vi "acquireSpectraWithOverSaturationProtection.vi"(8 "error in (no error)":errorcluster, 9 "NumberOfAcquisitions (1)":i32=1, 10 "default_integration_time":i32, 11 "VISA_name":refnum<visa-resource-name>) -> (0 "error out":errorcluster, 2 "integration_time":i32, 3 "Spectrum":dbl[](array[numeric]))   [LabVIEW 2015]
uses:
  <instrlib>/Ocean Optics 2000 4000/Ocean Optics 2000 4000.lvlib
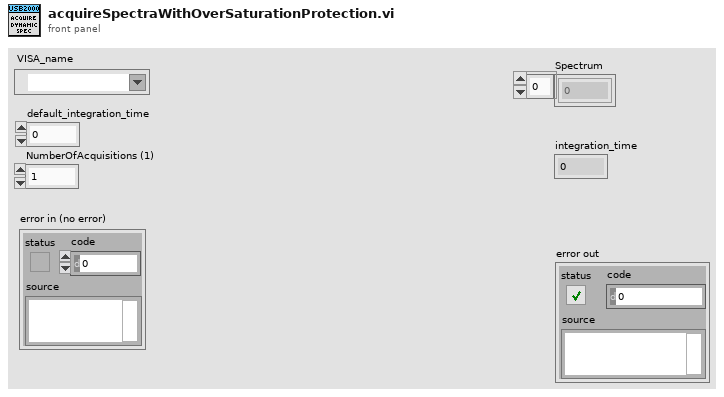
[diagram p1: front panel]
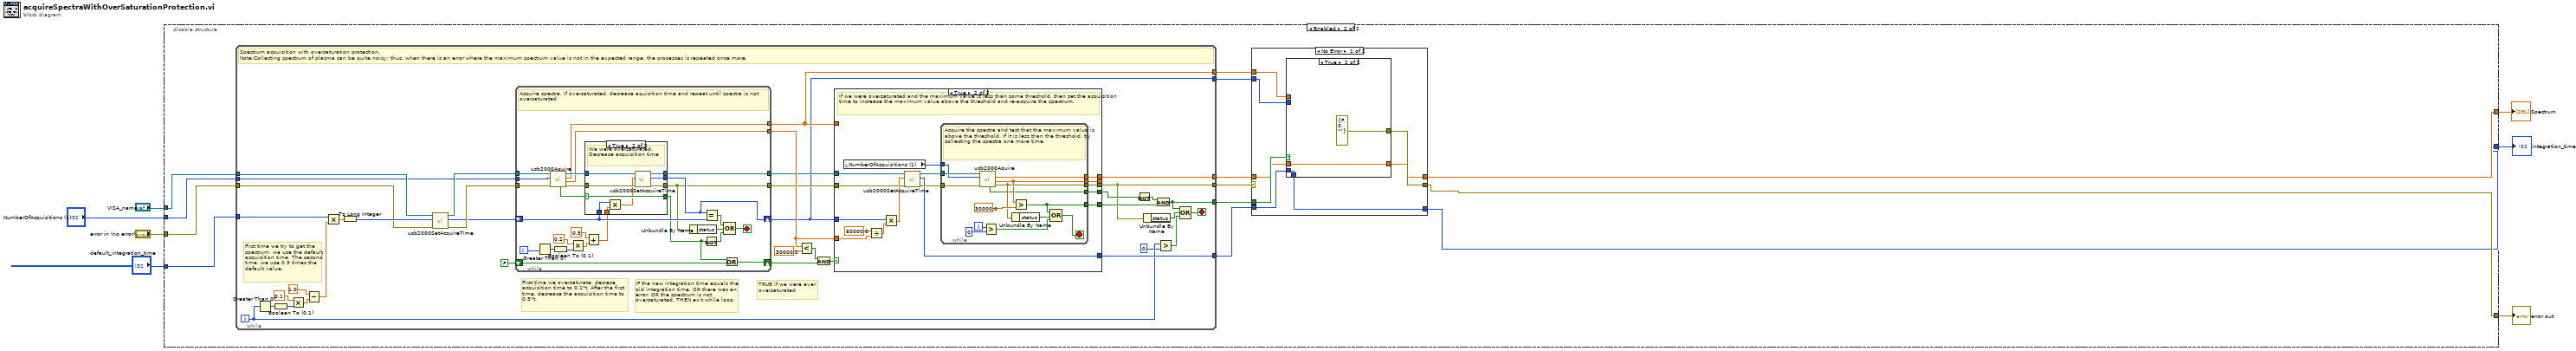
[diagram p0: block diagram]
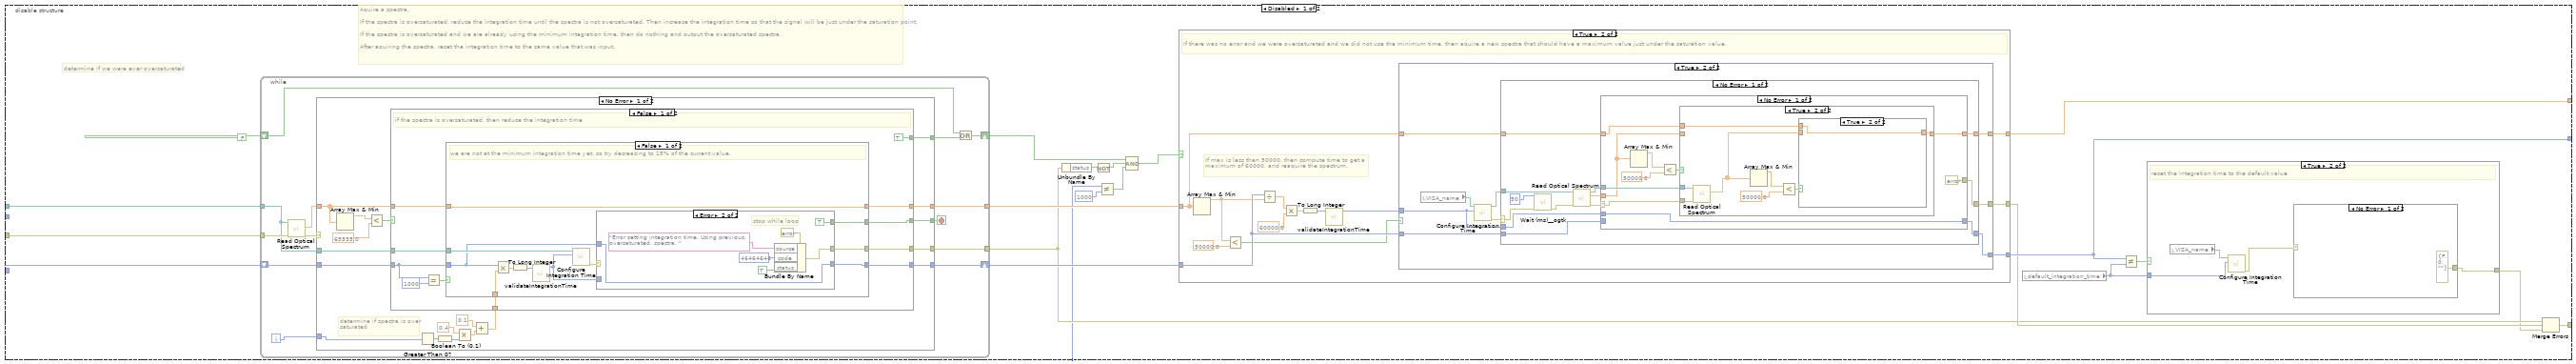
[diagram p2: hidden frame]
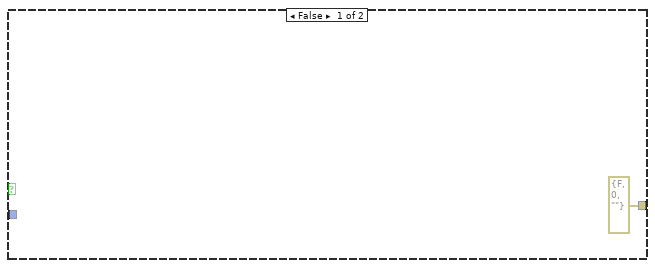
[diagram p3: hidden frame]
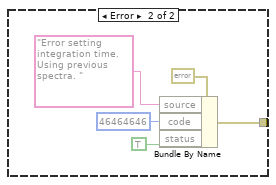
[diagram p4: hidden frame]
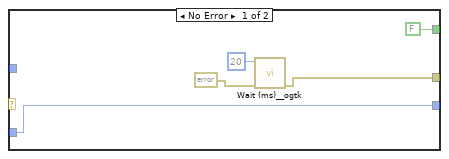
[diagram p5: hidden frame]
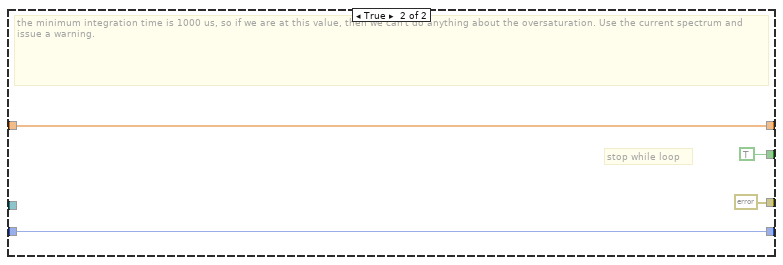
[diagram p6: hidden frame]
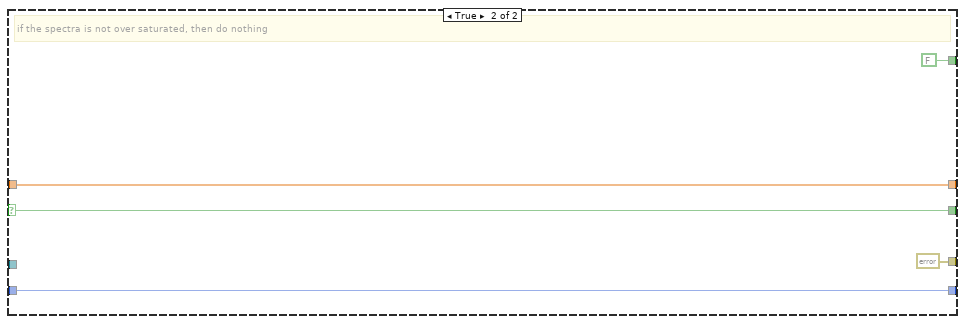
[diagram p7: hidden frame]
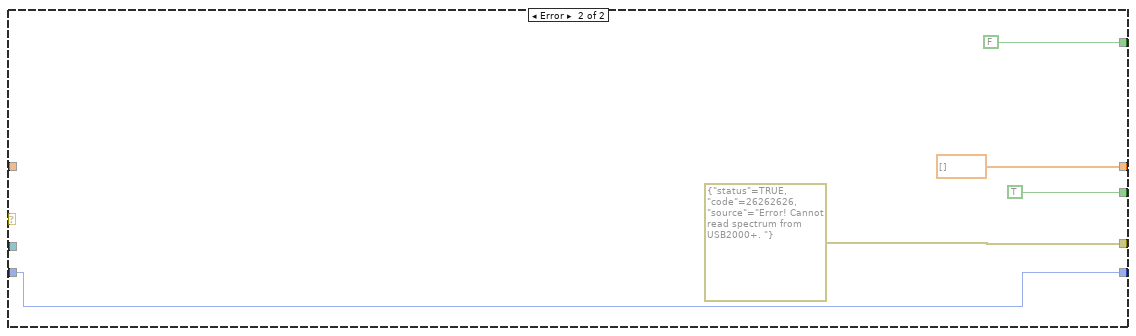
[diagram p8: hidden frame]
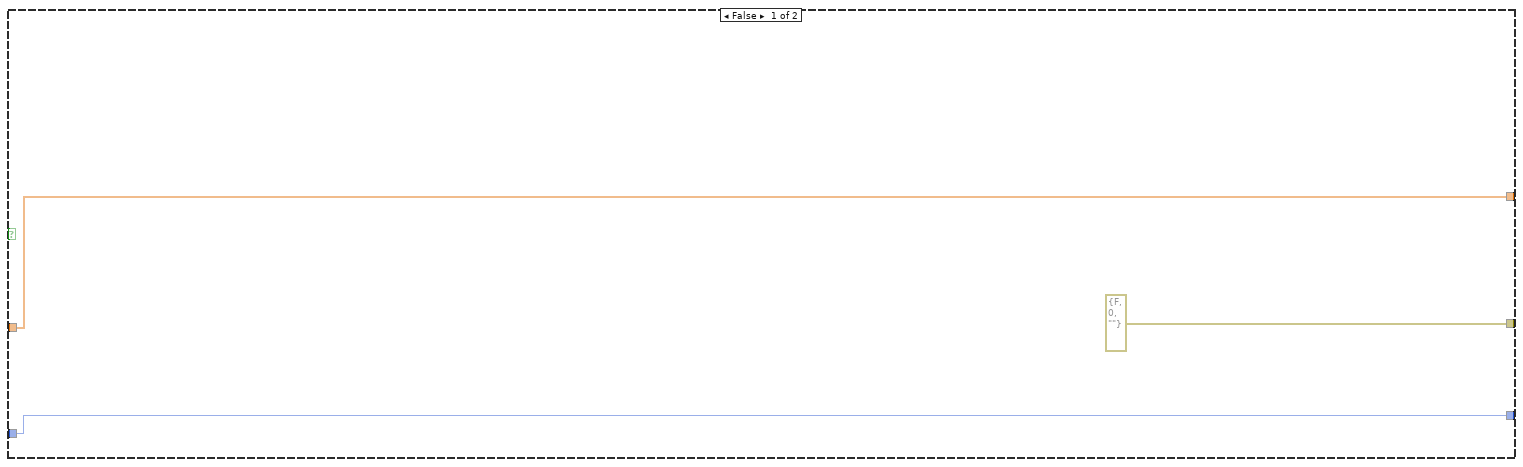
[diagram p9: hidden frame]
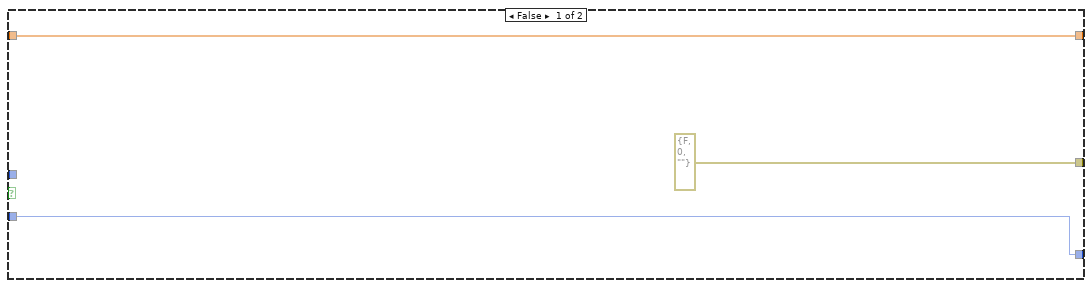
[diagram p10: hidden frame]
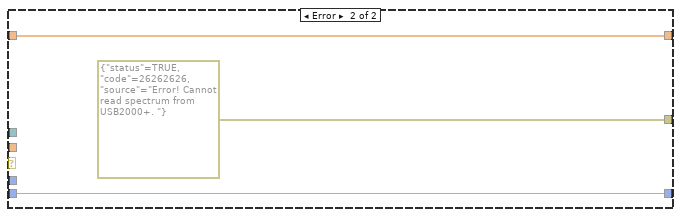
[diagram p13: hidden frame]
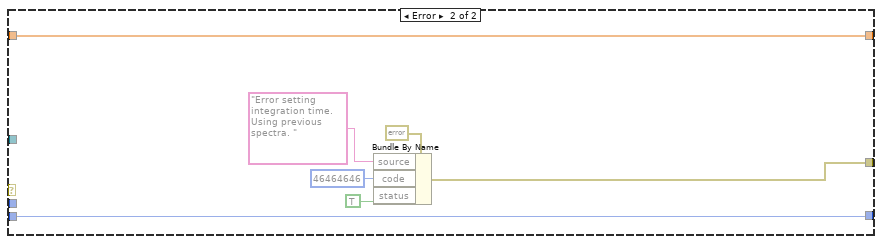
[diagram p14: hidden frame]
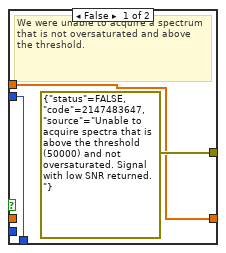
[diagram p15: hidden frame]
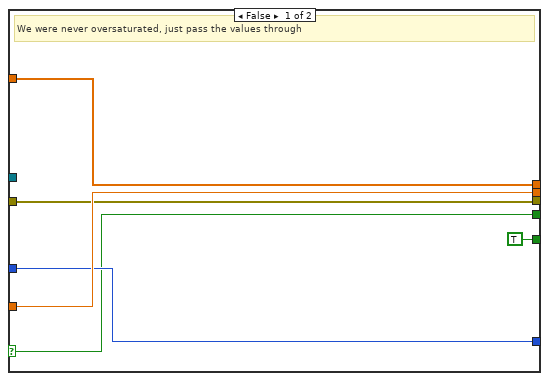
[diagram p17: hidden frame]
diagram:
  n1 = disable-structure shown="Enabled" {
    disable-tunnel: "error in (no error)" -> [w27 w198]
    disable-tunnel: [w19 w192] -> w6
    disable-tunnel: [w15 w194] -> w5
    disable-tunnel: [w14 w196] -> w4
    disable-tunnel: "default_integration_time" -> [w9 w199]
    disable-tunnel: "VISA_name" -> [w8 w197]
    disable-tunnel: "NumberOfAcquisitions (1)" -> [_ w195]
    frame Disabled {
      # "Aquire a spectra.\n\nIf the spectra is oversaturated, reduce the integration time until the spectra is not oversaturated. Then increase the integration time so that the signal will be just under the saturation point.\n\nIf the spectra is oversaturated and we are already using the minimum integration time, then do nothing and output the oversaturated spectra.\n\nAfter aquiring the spectra, reset the integration time to the same value that was input."
      # "determine if we were ever oversaturated"
      n2 = while {
        tunnel: w27 -> [w41]
        tunnel: w8 -> [w40]
        shift-right: [w49] -> w24
        shift-left: FALSE -> [w45]
        shift-right: [w48] -> w21
        shift-left: w9 -> [w51]
        tunnel: [w47] -> w20
        tunnel: [w44] -> w13
        i -> [w43]
        stop <- w50 stop-if-true
        n3 = call <instrlib>:"Read Optical Spectrum.vi"("error in (no error)"=w41, "VISA resource name"=w40) -> ("error out"=w39:errorcluster, "Spectrum by Pixels"=w42:dbl[])  [unwired: 6 in, 2 out]
        n4 = case shown="No Error" w39 {
          tunnel: w42 -> [w61 _]
          tunnel: [w62 errorcluster {"status"=TRUE, "code"=26262626, "source"="Error! Cannot read spectrum from USB2000+. "} ("error constant")] -> w44
          tunnel: [w68 dbl[] [] ("Spectrum by Pixels")] -> w47
          tunnel: w51 -> [w67 w115]
          tunnel: [w66 w115] -> w48
          tunnel: w40 -> [w65 _]
          tunnel: [w64 TRUE] -> w50
          tunnel: [w63 FALSE] -> w46
          tunnel: w43 -> [w58 _]
          frame No Error {
            # "determine if spectra is over saturated"
            n5 = Array Max & Min(array=w61) -> (max value=w60:dbl)  [unwired: 3 out]
            n6 = Less?(x=w60, y=65535.0) -> (x < y?=w59:bool)
            n7 = Greater Than 0?(x=w58) -> (x > 0?=w57:bool)
            n8 = Boolean To (0,1)(Boolean=w57) -> (0, 1=w56:i16)
            n9 = Multiply(x=0.4, y=w56) -> (x*y=w54:dbl)
            n10 = Add(x=0.1, y=w54) -> (x+y=w52:dbl)
            n11 = case shown="False" w59 {
              selector: w59 -> [_ w111]
              tunnel: w61 -> [w80 w112]
              tunnel: [w79 w112] -> w68
              tunnel: w67 -> [w72 w109]
              tunnel: [w78 w109] -> w66
              tunnel: w65 -> [w75 _]
              tunnel: [w77 w111] -> w64
              tunnel: [TRUE FALSE] -> w63
              tunnel: [w74 errorcluster {"status"=FALSE, "code"=0, "source"=""} ("error constant")] -> w62
              tunnel: w52 -> [w70 _]
              frame False {
                # "if the spectra is oversaturated, then reduce the integration time"
                n12 = Equal?(x=w72, y=1000) -> (x = y?=w73:bool)
                n13 = case shown="False" w73 {
                  tunnel: w80 -> [w89 w107]
                  tunnel: [w89 w107] -> w79
                  tunnel: w72 -> [w85 w106]
                  tunnel: [w86 w106] -> w78
                  tunnel: [w87 TRUE] -> w77
                  tunnel: w75 -> [w90 _]
                  tunnel: [w84 errorcluster {"status"=FALSE, "code"=0, "source"=""} ("error constant")] -> w74
                  tunnel: w70 -> [w81 _]
                  frame False {
                    # "we are not at the minimum integration time yet, so try decreasing to 15% of the current value."
                    n14 = Multiply(x=w85, y=w81) -> (x*y=w91:dbl)
                    n15 = To Long Integer(number=w91) -> (32bit integer=w83:i32)
                    n16 = call "validateIntegrationTime.vi"("integrationTime"=w83) -> ("validIntegrationTime"=w82:i32)  [unwired: 10 in]
                    n17 = call <instrlib>:"Configure Integration Time.vi"("Integration Time (6000)"=w82, "VISA resource name"=w90) -> ("error out"=w88:errorcluster)  [unwired: 1 in, 8 out]
                    n18 = case shown="Error" w88 {
                      tunnel: [FALSE TRUE] -> w87
                      tunnel: w82 -> [w95 _]
                      tunnel: [w95 w98] -> w86
                      tunnel: w85 -> [_ w98]
                      tunnel: [w93 w100] -> w84
                      frame No Error {
                        n19 = call <userlib>:"Wait (ms)__ogtk.vi"("error in (no error)"=errorcluster {"status"=FALSE, "code"=0, "source"=""} ("error constant"), "milliseconds to wait"=u32 20) -> ("error out"=w93:errorcluster)  [unwired: 8 in, 1 out]
                      }
                      frame Error {
                        # "stop while loop"
                        n20 = Bundle By Name(cluster=errorcluster {"status"=FALSE, "code"=0, "source"=""} ("error constant"), "source"="Error setting integration time. Using previous, oversaturated, spectra. ", "code"=46464646, "status"=TRUE) -> (w100:errorcluster)
                      }
                    }
                  }
                  frame True {
                    # "stop while loop"
                    # "the minimum integration time is 1000 us, so if we are at this value, then we can't do anything about the oversaturation. Use the current spectrum and issue a warning."
                  }
                }
              }
              frame True {
                # "if the spectra is not over saturated, then do nothing"
              }
            }
          }
          frame Error {
          }
        }
        n21 = Or(x=w45, y=w46) -> (x .or. y?=w49:bool)
      }
      n22 = Unbundle By Name(w13) -> ("status"=w25:bool)
      n23 = Not(x=w25) -> (.not. x?=w23:bool)
      n24 = Not Equal?(x=w9, y=1000) -> (x != y?=w10:bool)
      n25 = Compound Arithmetic op=AND(w24, w23, w10) -> (w22:bool)
      n26 = case shown="True" w22 {
        tunnel: w21 -> [w119 w128]
        tunnel: w20 -> [w120 w131]
        tunnel: [w120 w130] -> w14
        tunnel: [w119 w129] -> w19
        tunnel: [errorcluster {"status"=FALSE, "code"=0, "source"=""} ("error constant") w127] -> w16
        frame False {
        }
        frame True {
          # "If max is less than 50000, then compute time to get a maximum of 60000, and reaquire the spectrum."
          # "If there was no error and we were oversaturated and we did not use the minimum time, then aquire a new spectra that should have a maximum value just under the saturation value."
          n27 = Array Max & Min(array=w131) -> (max value=w123:dbl)  [unwired: 3 out]
          n28 = Less?(x=w123, y=50000.0) -> (x < y?=w121:bool)
          n29 = Divide(x=w128, y=w123) -> (x/y=w133:dbl)
          n30 = Multiply(x=w133, y=60000.0) -> (x*y=w132:dbl)
          n31 = To Long Integer(number=w132) -> (32bit integer=w125:i32)
          n32 = call "validateIntegrationTime.vi"("integrationTime"=w125) -> ("validIntegrationTime"=w124:i32)  [unwired: 10 in]
          n33 = case shown="True" w121 {
            tunnel: w124 -> [_ w139]
            tunnel: w131 -> [w136 w143]
            tunnel: [w136 w142] -> w130
            tunnel: [w135 w140] -> w129
            tunnel: w128 -> [w135 w137]
            tunnel: [errorcluster {"status"=FALSE, "code"=0, "source"=""} ("error constant") w141] -> w127
            frame False {
            }
            frame True {
              n34 = local read "VISA_name"() -> (w144:refnum<visa-resource-name>)
              n35 = call <instrlib>:"Configure Integration Time.vi"("Integration Time (6000)"=w139, "VISA resource name"=w144) -> ("error out"=w145:errorcluster, "VISA resource name out"=w138:refnum<visa-resource-name>)  [unwired: 1 in, 7 out]
              n36 = case shown="No Error" w145 {
                selector: w145 -> [w152 _]
                tunnel: [w156 w187] -> w141
                tunnel: w138 -> [w150 _]
                tunnel: w143 -> [w157 w184]
                tunnel: [w158 w184] -> w142
                tunnel: w139 -> [w155 _]
                tunnel: [w153 w183] -> w140
                tunnel: w137 -> [w154 w183]
                frame No Error {
                  n37 = call <userlib>:"Wait (ms)__ogtk.vi"("error in (no error)"=w152, "milliseconds to wait"=u32 50) -> ("error out"=w149:errorcluster)  [unwired: 8 in, 1 out]
                  n38 = call <instrlib>:"Read Optical Spectrum.vi"("error in (no error)"=w149, "VISA resource name"=w150) -> ("error out"=w147:errorcluster, "Spectrum by Pixels"=w148:dbl[], "VISA resource name out"=w146:refnum<visa-resource-name>)  [unwired: 6 in, 1 out]
                  n39 = case shown="No Error" w147 {
                    selector: w147 -> [w163 _]
                    tunnel: w148 -> [w161 _]
                    tunnel: [w160 w182] -> w158
                    tunnel: w157 -> [w159 w182]
                    tunnel: [errorcluster {"status"=FALSE, "code"=0, "source"=""} ("error constant") errorcluster {"status"=TRUE, "code"=26262626, "source"="Error! Cannot read spectrum from USB2000+. "} ("error constant")] -> w156
                    tunnel: w155 -> [w167 _]
                    tunnel: w154 -> [_ w180]
                    tunnel: [w167 w180] -> w153
                    tunnel: w146 -> [w162 _]
                    frame No Error {
                      n40 = Array Max & Min(array=w161) -> (max value=w166:dbl)  [unwired: 3 out]
                      n41 = Less?(x=w166, y=50000.0) -> (x < y?=w164:bool)
                      n42 = case shown="True" w164 {
                        tunnel: w163 -> [_ w177]
                        tunnel: w162 -> [_ w176]
                        tunnel: w161 -> [w169 _]
                        tunnel: [w169 w171] -> w160
                        tunnel: w159 -> [_ w170]
                        frame False {
                        }
                        frame True {
                          n43 = call <instrlib>:"Read Optical Spectrum.vi"("error in (no error)"=w177, "VISA resource name"=w176) -> ("Spectrum by Pixels"=w172:dbl[])  [unwired: 6 in, 3 out]
                          n44 = Array Max & Min(array=w172) -> (max value=w174:dbl)  [unwired: 3 out]
                          n45 = Less?(x=w174, y=50000.0) -> (x < y?=w173:bool)
                          n46 = case shown="True" w173 {
                            tunnel: w172 -> [w178 _]
                            tunnel: [w178 w179] -> w171
                            tunnel: w170 -> [_ w179]
                            frame False {
                            }
                            frame True {
                            }
                          }
                        }
                      }
                    }
                    frame Error {
                    }
                  }
                }
                frame Error {
                  n47 = Bundle By Name(cluster=errorcluster {"status"=FALSE, "code"=0, "source"=""} ("error constant"), "source"="Error setting integration time. Using previous spectra. ", "code"=46464646, "status"=TRUE) -> (w187:errorcluster)
                }
              }
            }
          }
        }
      }
      n48 = local read "default_integration_time"() -> (w17:i32)
      n49 = Not Equal?(x=w19, y=w17) -> (x != y?=w18:bool)
      n50 = case shown="True" w18 {
        tunnel: w17 -> [_ w31]
        tunnel: [errorcluster {"status"=FALSE, "code"=0, "source"=""} ("error constant") w29] -> w12
        frame False {
        }
        frame True {
          # "reset the integration time to the default value"
          n51 = local read "VISA_name"() -> (w32:refnum<visa-resource-name>)
          n52 = call <instrlib>:"Configure Integration Time.vi"("Integration Time (6000)"=w31, "VISA resource name"=w32) -> ("error out"=w30:errorcluster)  [unwired: 1 in, 8 out]
          n53 = case shown="No Error" w30 {
            tunnel: [errorcluster {"status"=FALSE, "code"=0, "source"=""} ("error constant") w34] -> w29
            frame No Error {
            }
            frame Error {
              n54 = Bundle By Name(cluster=errorcluster {"status"=FALSE, "code"=0, "source"=""} ("error constant"), "source"="Error setting integration time. Using previous spectra. ", "code"=46464646, "status"=TRUE) -> (w34:errorcluster)
            }
          }
        }
      }
      n55 = Merge Errors(w13, w16, w12) -> (w15:errorcluster)
    }
    frame Enabled {
      n56 = while {
        tunnel: w199 -> [w233]
        tunnel: [w241] -> w202
        tunnel: [w240] -> w200
        tunnel: [w239] -> w193
        tunnel: [w231] -> w201
        tunnel: w197 -> [w224]
        tunnel: w198 -> [w223]
        tunnel: w195 -> [w222]
        tunnel: [w221] -> w191
        tunnel: [w220] -> w190
        i -> [w234]
        stop <- w242 stop-if-true
        # "First time we try to get the spectrum, we use the default acquisition time. The second time, we use 0.9 times the default value."
        # "IF the new integration time equals the old integration time, OR there was an error, OR the spectrum is not oversaturated, THEN exit while loop"
        # "First time we oversaturate, decrese acquisition time to 0.1*t. After the first time, decrease the acquisition time to 0.5*t."
        # "TRUE if we were ever oversaturated"
        # "Spectrum acquisition with oversaturation protection. \nNote:Collecting spectrum of plasma can be quite noisy; thus, when there is an error where the maximum spectrum value is not in the expected range, the processes is repeated once more."
        n57 = Greater Than 0?(x=w234) -> (x > 0?=w229:bool)
        n58 = Boolean To (0,1)(Boolean=w229) -> (0, 1=w238:i16)
        n59 = Multiply(x=0.1, y=w238) -> (x*y=w236:dbl)
        n60 = Subtract(x=1.0, y=w236) -> (x-y=w232:dbl)
        n61 = Multiply(x=w233, y=w232) -> (x*y=w230:dbl)
        n62 = To Long Integer(number=w230) -> (32bit integer=w225:i32)
        n63 = call "usb2000SetAcquireTime.vi"("error in (no error)"=w223, "Integration Time (6000)"=w225, "VISA resource name"=w224) -> ("error out"=w227:errorcluster, "validIntegrationTime"=w226:i32, "VISA resource name out"=w228:refnum<visa-resource-name>)  [unwired: 6 in]
        n64 = while {
          shift-right: [w303] -> w220
          shift-left: w226 -> [w309]
          tunnel: [w302] -> w221
          tunnel: [w301] -> w251
          shift-right: [w300] -> w252
          shift-left: FALSE -> [w298]
          tunnel: [w297] -> w250
          tunnel: [w296] -> w249
          tunnel: w228 -> [w295]
          tunnel: w227 -> [w294]
          tunnel: w222 -> [w293]
          i -> [w310]
          stop <- w304 stop-if-true
          # "Acquire spectra. If oversaturated, decrease aquisition time and repeat until spectra is not oversaturated"
          n65 = Greater Than 0?(x=w310) -> (x > 0?=w311:bool)
          n66 = call "usb2000Aquire.vi"("error in (no error)"=w294, "NumberOfAcquisitions (1)"=w293, "VISA resource name"=w295) -> ("error out"=w317:errorcluster, "MaxValue"=w301:dbl, "Spectrum by Pixels"=w302:dbl[], "VISA resource name out"=w316:refnum<visa-resource-name>, "oversaturated"=w318:bool)  [unwired: 4 in]
          n67 = Boolean To (0,1)(Boolean=w311) -> (0, 1=w312:i16)
          n68 = Multiply(x=0.2, y=w312) -> (x*y=w314:dbl)
          n69 = Add(x=0.5, y=w314) -> (x+y=w308:dbl)
          n70 = case shown="True" w318 {
            selector: w318 -> [w322 w328]
            tunnel: w317 -> [w321 w331]
            tunnel: w316 -> [w319 w330]
            tunnel: [w321 w329] -> w297
            tunnel: [w322 w328] -> w299
            tunnel: [w320 w327] -> w303
            tunnel: w309 -> [w320 w326]
            tunnel: w308 -> [_ w325]
            tunnel: [w319 w323] -> w296
            frame False {
            }
            frame True {
              # "We were oversaturated. Decrease acquisition time"
              n71 = Multiply(x=w326, y=w325) -> (x*y=w324:dbl)
              n72 = call "usb2000SetAcquireTime.vi"("error in (no error)"=w331, "Integration Time (6000)"=w324, "VISA resource name"=w330) -> ("error out"=w329:errorcluster, "validIntegrationTime"=w327:i32, "VISA resource name out"=w323:refnum<visa-resource-name>)  [unwired: 6 in]
            }
          }
          n73 = Unbundle By Name(w297) -> ("status"=w306:bool)
          n74 = Not(x=w299) -> (.not. x?=w305:bool)
          n75 = Equal?(x=w303, y=w309) -> (x = y?=w307:bool)
          n76 = Compound Arithmetic op=OR(w307, w306, w305) -> (w304:bool)
          n77 = Or(x=w299, y=w298) -> (x .or. y?=w300:bool)
        }
        n78 = Less?(x=w251, y=30000.0) -> (x < y?=w253:bool)
        n79 = And(x=w253, y=w252) -> (x .and. y?=w254:bool)
        n80 = case shown="True" w254 {
          selector: w254 -> [w257 _]
          tunnel: w220 -> [w259 w278]
          tunnel: w251 -> [w261 w275]
          tunnel: w250 -> [w260 w274]
          tunnel: w249 -> [_ w272]
          tunnel: [w259 w269] -> w239
          tunnel: [w260 w266] -> w240
          tunnel: [w261 w268] -> _
          tunnel: [w262 w267] -> w241
          tunnel: w221 -> [w262 _]
          tunnel: [w257 w265] -> w245
          tunnel: [TRUE w264] -> w246
          frame False {
            # "We were never oversaturated, just pass the values through"
          }
          frame True {
            # "If we were oversaturated and the maximum value is less than some threshold, then set the acquisition time to increase the maximum value above the threshold and re-acquire the spectrum."
            n81 = local read "NumberOfAcquisitions (1)"() -> (w263:i32)
            n82 = Divide(x=60000.0, y=w275) -> (x/y=w277:dbl)
            n83 = Multiply(x=w278, y=w277) -> (x*y=w273:dbl)
            n84 = call "usb2000SetAcquireTime.vi"("error in (no error)"=w274, "Integration Time (6000)"=w273, "VISA resource name"=w272) -> ("error out"=w271:errorcluster, "validIntegrationTime"=w269:i32, "VISA resource name out"=w270:refnum<visa-resource-name>)  [unwired: 6 in]
            n85 = while {
              tunnel: w271 -> [w292]
              tunnel: w270 -> [w291]
              tunnel: [w287] -> w267
              tunnel: [w283] -> w266
              tunnel: [w282] -> w268
              tunnel: [w281] -> w265
              tunnel: [w280] -> w264
              tunnel: w263 -> [w279]
              i -> [w289]
              stop <- w284 stop-if-true
              # "Acquire the spectra and test that the maximum value is above the threshold. If it is less than the threshold, try collecting the spectra one more time."
              n86 = call "usb2000Aquire.vi"("error in (no error)"=w292, "NumberOfAcquisitions (1)"=w279, "VISA resource name"=w291) -> ("error out"=w283:errorcluster, "MaxValue"=w282:dbl, "Spectrum by Pixels"=w287:dbl[], "oversaturated"=w281:bool)  [unwired: 4 in, 1 out]
              n87 = Greater?(x=w289, y=0) -> (0:w285:bool)
              n88 = Unbundle By Name(w283) -> ("status"=w286:bool)
              n89 = Greater?(x=w282, y=30000.0) -> (0:w280:bool)
              n90 = Compound Arithmetic op=OR(w280, w286, w285) -> (w284:bool)
            }
          }
        }
        n91 = Not(x=w245) -> (.not. x?=w247:bool)
        n92 = Unbundle By Name(w240) -> ("status"=w248:bool)
        n93 = And(x=w247, y=w246) -> (x .and. y?=w231:bool)
        n94 = Greater?(x=w234, y=0) -> (0:w243:bool)
        n95 = Compound Arithmetic op=OR(w231, w248, w243) -> (w242:bool)
      }
      n96 = case shown="No Error" w200 {
        selector: w200 -> [_ w217]
        tunnel: w201 -> [w210 _]
        tunnel: [w209 w217] -> w194
        tunnel: w202 -> [w204 _]
        tunnel: [w206 w219] -> w196
        tunnel: w193 -> [w203 _]
        tunnel: [w205 w218] -> w192
        tunnel: w191 -> [w208 w219]
        tunnel: w190 -> [w207 w218]
        frame No Error {
          n97 = case shown="True" w210 {
            tunnel: [errorcluster {"status"=FALSE, "code"=2147483647, "source"="Unable to acquire spectra that is above the threshold (50000) and not oversaturated. Signal with low SNR returned."} ("error constant") errorcluster {"status"=FALSE, "code"=0, "source"=""} ("error constant")] -> w209
            tunnel: w208 -> [w212 _]
            tunnel: w207 -> [w211 _]
            tunnel: [w212 w215] -> w206
            tunnel: [w211 w214] -> w205
            tunnel: w204 -> [_ w215]
            tunnel: w203 -> [_ w214]
            frame False {
              # "We were unable to acquire a spectrum that is not oversaturated and above the threshold."
            }
            frame True {
            }
          }
        }
        frame Error {
        }
      }
    }
  }
  "error out" <- w5
  "Spectrum" <- w4
  "integration_time" <- w6
